vi "Thorlab_MotorCtrl.vi"() -> ()   [LabVIEW 2016]
doc: "This VI contains a basic quadrature decoder which is reset asynchronously upon clicking the reset button."
uses:
  <vilib>/Platform/TimedLoop/XDataNode/timing_clust.ctl
  <vilib>/Platform/TimedLoop/XDataNode/nitl_modes.ctl
  <vilib>/Platform/TimedLoop/XDataNode/wakeup.ctl
  <vilib>/rvi/Emulation/niFpgaSctlEmulationGetInTimedLoop.vi
  <vilib>/rvi/Emulation/niFpgaEmulationReportErrorSimple.vi
  <vilib>/rvi/Emulation/niFpgaGetClockAttributes.vi
  <vilib>/rvi/Emulation/niFpgaCriticalErrorInLSC.vi
  <vilib>/platform/TimedLoop/XDataNode/XDataNode.xnode
  <vilib>/Platform/TimedLoop/XDataNode/XDNodeRunTimeDep.lvlib
  Library/jmslib.lvlib
panel:
  in  "DIR Y":bool
  in  "INHB Y":bool
  out "FAULT Y":bool
  out "Position Y":i32
  out "JumpBy2Error Y":i16
  in  "Reset Y":bool
  in  "Y DC":fxp<+,32,0>
  out "samples":i32
  out "Current Monitor":u32[](array[numeric])
  out "Raw Data Response (MSB)":bool[](array[boolean])
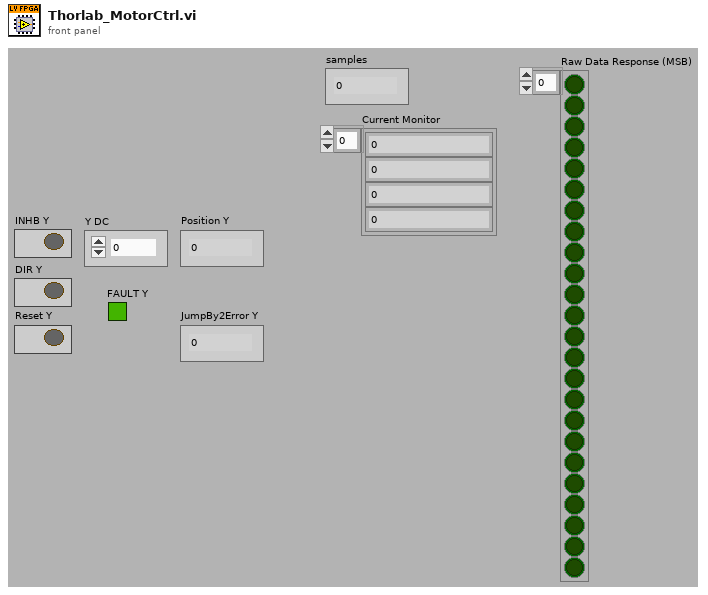
[diagram p1: front panel]
types:
  T1 = typedef "XDNodeRunTimeDep.lvlib/timing_clust.ctl" = cluster{"Expected End [f-1]":u64, "Actual End [f-1]":u64, "Finished Late? [f-1]":bool, "Expected End [i-1]":u64, "Actual End [i-1]":u64, "Finished Late? [i-1]":bool, "Expected Start [i]":u64, "Actual Start [i]":u64, "Expected Start [f]":u64, "Actual Start [f]":u64, "Source Name":string, "Structure Name":string, "Period":i64, "Deadline":i64, "Offset":i64, "Start":i64, "Priority":i32, "Timeout":i32, "Mode":T2, "Wakeup Reason":T3, "Error":errorcluster, "Source Type":string, "Secondary Source Type":string, "Global End Time":u64, "Global Start Time":u64, "Frame Duration":u64, "Iteration Duration":u64, "Assigned CPU":i32, "I/O Scan Engine Mode":u32}
  T2 = typedef "XDNodeRunTimeDep.lvlib/nitl_modes.ctl" = enum32{"No Change", "Process missed periods, maintain original phase", "Discard missed periods, maintain original phase", "Process missed periods, ignore original phase", "Discard missed periods, ignore original phase"}
  T3 = typedef "XDNodeRunTimeDep.lvlib/wakeup.ctl" = enum32{"Normal", "Aborted", "Asynchronous wakeup", "Timing source error", "Timed loop error", "Timeout"}
  T4 = cluster{"PWM In":refnum<k21>, "Direction":refnum<k21>, "Inhibit":refnum<k21>, "Encoder C":refnum<k21>, "Encoder B":refnum<k21>, "Encoder A":refnum<k21>, "Fault":refnum<k21>}
  T5 = cluster{"SCLK":refnum<k21>, "MOSI":refnum<k21>, "MISO":refnum<k21>}
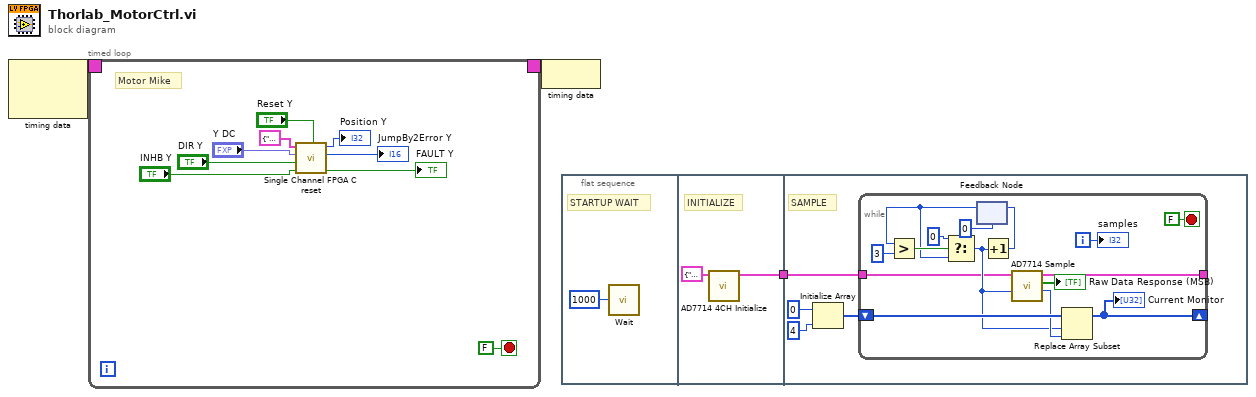
[diagram p0: block diagram]
diagram:
  n1 = node-c288() -> (w3:T1)  [unwired: 2 in]
  n2 = timed-loop {
    timing: w3 -> [_]
    timing-out: [_] -> w2
    stop <- FALSE stop-if-true
    # "Motor Mike"
    n3 = call "Single Channel FPGA C reset.vi"("Reset"="Reset Y", "INHB"="INHB Y", "DIR"="DIR Y", "Duty"="Y DC", "IO Channels"=T4 {"PWM In"="Connector1/DIO1", "Direction"="Connector1/DIO2", "Inhibit"="Connector1/DIO3", "Encoder C"="Connector1/DIO4", "Encoder B"="Connector1/DIO5", "Encoder A"="Connector1/DIO6", "Fault"="Connector1/DIO0"}) -> ("FAULT"=→"FAULT Y":bool, "JumpBy2Error"=→"JumpBy2Error Y":i16, "Position"=→"Position Y":i32)  [unwired: 4 in]
  }
  n4 = node-c288(w2) -> ()
  n5 = flat-sequence {
    tunnel: [w16] -> w1
    tunnel: w1 -> [w18]
    frame #0 {
      # "STARTUP WAIT"
      n6 = call "Wait"("Count(uSec)"=u32 1000) -> ()  [unwired: 1 out]
    }
    frame #1 {
      # "INITIALIZE"
      n7 = call "AD7714 4CH Initialize.vi"("I/O Cluster In"=T5 {"SCLK"="Connector1/DIO29", "MOSI"="Connector1/DIO35", "MISO"="Connector1/DIO31"}) -> ("I/O Cluster Out"=w16:T5)  [unwired: 10 in]
    }
    frame #2 {
      # "SAMPLE"
      n8 = Initialize Array(u32 0, 4 ("dimension size")) -> (w19:u32[])
      n9 = while {
        shift-right: [w27] -> _
        shift-left: w19 -> [w28]
        tunnel: w18 -> [w24]
        tunnel: [w23] -> _
        i -> [w35]
        stop <- FALSE stop-if-true
        n10 = feedback #1(i16 0) -> (w31:i16)
        n11 = Greater?(x=w31, y=i16 3) -> (0:w32:bool)
        n12 = Select(t=i16 0, s=w32, f=w31) -> (s? t:f=w25:i16)
        n13 = Increment(x=w25) -> (x+1=w29:i16)
        n14 = feedback-in #1(w29) -> ()
        n15 = call "AD7714 Sample.vi"("Channel"=w25, "I/O Cluster In"=w24) -> ("Data"=w26:u32, "Raw Data Response (MSB)"=→"Raw Data Response (MSB)":bool[], "I/O Cluster Out"=w23:T5)  [unwired: 7 in]
        n16 = Replace Array Subset(array=w28, new element=w26, index=w25) -> (w27:u32[])
        "Current Monitor" <- w27
        "samples" <- w35
      }
    }
  }
